vi "SIMDMM_DU64_U32AddWithOverflow.vi"(2 "input 2":u32, 3 "input 1":u32) -> (0 "output":u32, 1 "overflow":u32)   [LabVIEW 2019]
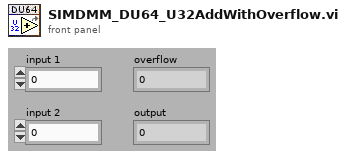
[diagram p1: front panel]
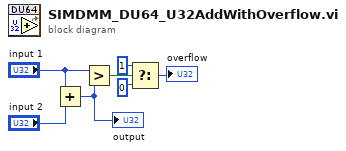
[diagram p0: block diagram]
diagram:
  n1 = Add(x="input 1", y="input 2") -> (x+y=w6:u32)
  "output" <- w6
  n2 = Greater?(x="input 1", y=w6) -> (0:w3:bool)
  n3 = Select(t=u32 1 ("output"), s=w3, f=u32 0 ("output")) -> (s? t:f=→"overflow":u32)
